vi "AlliGator Get Series Subfolders Information.vi"(8 "error in (no error)":errorcluster, 10 "pattern":string, 11 "Path":path) -> (0 "error out":errorcluster, 1 "Subfolder Paths":path[](array[path]), 2 "Sorted Subfolder Names":string[](array[string]), 3 "dup directory path":path, 4 "# Files":i32[](array[numeric]), 5 "Files in the Root Folder":string[](array[string]), 6 "Same # Files?":bool)   [LabVIEW 2021, in "AlliGator Scripts.lvlib"]
doc: "Returns a breadown of the folder's content for subsequent script actions."
uses:
  AlliGator Scripts.lvlib
  <userlib>/_OpenG.lib/file/file.llb/openg_file.lvlib
  Strings/Strings.lvlib
panel:
  # "see the AlliGator License on the block diagram (Ctrl+E or Window:Show Block Diagram)"
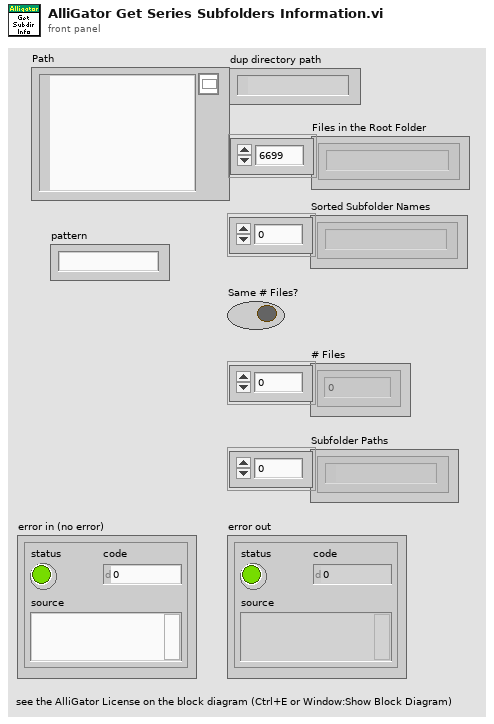
[diagram p1: front panel]
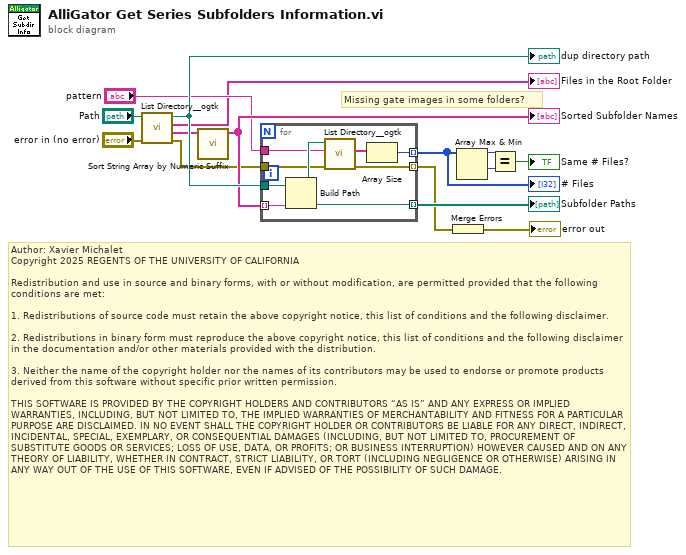
[diagram p0: block diagram]
diagram:
  # "Author: Xavier Michalet\nCopyright 2025 REGENTS OF THE UNIVERSITY OF CALIFORNIA\n\nRedistribution and use in source and binary forms, with or without modification, are permitted provided that the following conditions are met:\n\n1. Redistributions of source code must retain the above copyright notice, this list of conditions and the following disclaimer.\n\n2. Redistributions in binary form must reproduce the above copyright notice, this list of conditions and the following disclaimer in the documentation and/or other materials provided with the distribution.\n\n3. Neither the name of the copyright holder nor the names of its contributors may be used to endorse or promote products derived from this software without specific prior written permission.\n\nTHIS SOFTWARE IS PROVIDED BY THE COPYRIGHT HOLDERS AND CONTRIBUTORS “AS IS” AND ANY EXPRESS OR IMPLIED WARRANTIES, INCLUDING, BUT NOT LIMITED TO, THE IMPLIED WARRANTIES OF MERCHANTABILITY AND FITNESS FOR A PARTICULAR PURPOSE ARE DISCLAIMED. IN NO EVENT SHALL THE COPYRIGHT HOLDER OR CONTRIBUTORS BE LIABLE FOR ANY DIRECT, INDIRECT, INCIDENTAL, SPECIAL, EXEMPLARY, OR CONSEQUENTIAL DAMAGES (INCLUDING, BUT NOT LIMITED TO, PROCUREMENT OF SUBSTITUTE GOODS OR SERVICES; LOSS OF USE, DATA, OR PROFITS; OR BUSINESS INTERRUPTION) HOWEVER CAUSED AND ON ANY THEORY OF LIABILITY, WHETHER IN CONTRACT, STRICT LIABILITY, OR TORT (INCLUDING NEGLIGENCE OR OTHERWISE) ARISING IN ANY WAY OUT OF THE USE OF THIS SOFTWARE, EVEN IF ADVISED OF THE POSSIBILITY OF SUCH DAMAGE."
  # "Missing gate images in some folders?"
  n1 = call <userlib>:"List Directory__ogtk.vi"("error in (no error)"="error in (no error)", "directory path"="Path") -> ("error out"=w3:errorcluster, "directory names"=w13:string[], "file names"=→"Files in the Root Folder":string[], "dup directory path"=w15:path)  [unwired: 2 in]
  "dup directory path" <- w15
  n2 = call "Sort String Array by Numeric Suffix.vi"("String Array"=w13) -> ("Sorted String Array"=w14:string[])  [unwired: 8 in, 2 out]
  "Sorted Subfolder Names" <- w14
  n3 = for {
    tunnel: w14 -> [w23] mode=indexing
    tunnel: w15 -> [w22]
    tunnel: [w20] -> w4 mode=indexing
    tunnel: [w19] -> w12 mode=indexing
    tunnel: "pattern" -> [w18]
    tunnel: w3 -> [w17]
    tunnel: [w16] -> w2 mode=indexing
    n4 = Build Path(base path=w22, name or relative path=w23) -> (appended path=w20:path)
    n5 = call <userlib>:"List Directory__ogtk.vi"("error in (no error)"=w17, "pattern"=w18, "directory path"=w20) -> ("error out"=w16:errorcluster, "file names"=w21:string[])  [unwired: 1 in, 2 out]
    n6 = Array Size(array=w21) -> (size(s)=w19:i32)
  }
  "# Files" <- w12
  "Subfolder Paths" <- w4
  n7 = Merge Errors(w2) -> (→"error out":errorcluster)
  n8 = Array Max & Min(array=w12) -> (max value=w8:i32, min value=w6:i32)  [unwired: 2 out]
  n9 = Equal?(x=w8, y=w6) -> (x = y?=→"Same # Files?":bool)
